vi "量测站CT内容.vi"() -> (0 "tablename":string, 3 "data":string[](array[string]))   [LabVIEW 2017]
uses:
  Sqlite/CBB/ReadAllData.vi
  Sqlite/SQLite.lvlib
panel:
  out "大小 2":i32
  out "大小":i32
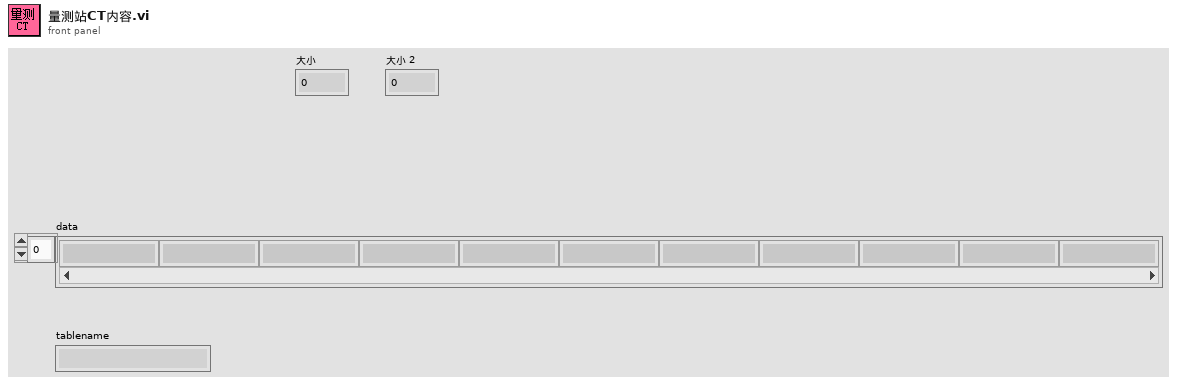
[diagram p1: front panel]
types:
  T1 = typedef "动子1&2CT操作选项.ctl" = enum16{"初始化", "出料轴接料", "投掷出料区", "获取寄存器", "更新等待CT"}
  T2 = typedef "动子3&4CT操作选项.ctl" = enum16{"初始化", "扫码+CheckRoute", "BK拍照", "BT+对位", "RT贴合", "Servo压合", "p400复检", "获取寄存器", "更新等待时间"}
  T3 = typedef "data格式选项.ctl" = enum16{"生成格式", "加载格式"}
  T4 = typedef "pathcheck选项.ctl" = enum16{"ProductData", "CTData", "ERData", "IOTDATA"}
  T5 = typedef "IOT time.ctl" = cluster{"Work":string, "Inflow":string, "Outflow":string, "Wait":string}
  T6 = typedef "上一次缓存.ctl" = cluster{"CT集合":string[], "in /out time":T7, "SN缓存":string}
  T7 = typedef "in_out time.ctl" = cluster{"input-time":string, "output-time":string, "wait-starttime":dbl, "wait-time":string}
  T8 = typedef "表头集合.ctl" = cluster{"product信息":T9, "CT信息":T10, "ER信息":T11, "IOT信息":T12}
  T9 = typedef "product信息.ctl" = cluster{"product表头整合":string[], "量测部分表头":string[], "前侧贴合表头":string[], "后侧贴合表头":string[]}
  T10 = typedef "CT信息.ctl" = cluster{"CT表头整合":string[], "量测CT":string[], "动子1_2CT":string[], "动子3_4CT":string[]}
  T11 = typedef "ER信息.ctl" = cluster{"ER表头整合":string[]}
  T12 = typedef "IOT信息.ctl" = cluster{"IOT表头整合":string[]}
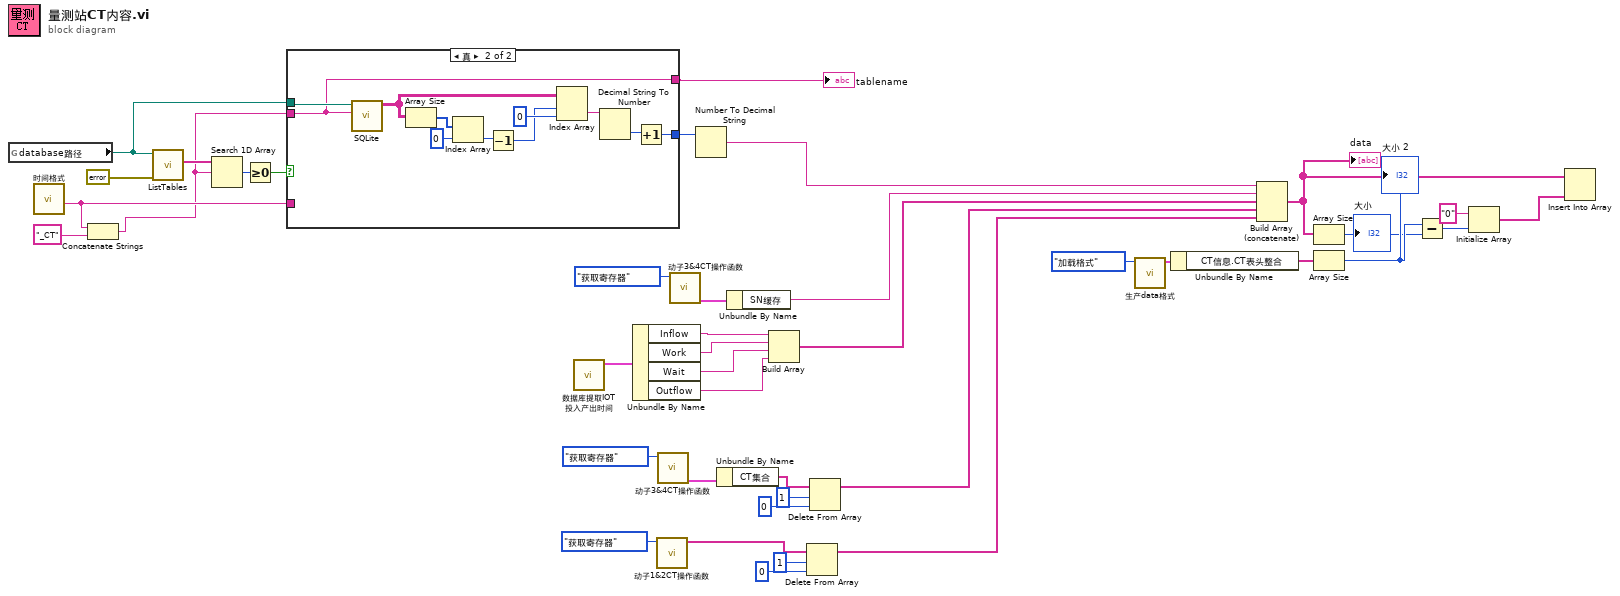
[diagram p0: block diagram]
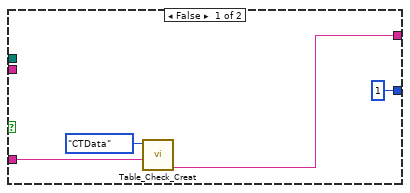
[diagram p2: hidden frame]
diagram:
  n1 = global read "数据库全局.vi" "database路径"() -> (w27:path)
  n2 = call "时间格式.vi"() -> ("_Date"=w25:string)  [unwired: 7 in, 4 out]
  n3 = Concatenate Strings(w25, "_CT" ("字符串")) -> (w24:string)
  n4 = call "ListTables.vi"("error in (no error)"=errorcluster {"status"=FALSE, "code"=0, "source"=""}, "DbPath"=w27) -> ("Tables"=w30:string[])  [unwired: 6 in, 3 out]
  n5 = Search 1D Array(1D array=w30, element=w24) -> (index of element=w31:i32)  [unwired: 1 in]
  n6 = Greater Or Equal To 0?(x=w31) -> (x >= 0?=w28:bool)
  n7 = case shown="真" w28 {
    tunnel: w27 -> [_ w55]
    tunnel: w24 -> [_ w45]
    tunnel: [1 w46] -> w26
    tunnel: w25 -> [w42 _]
    tunnel: [w41 w45] -> w23
    frame False {
      n8 = call "Table_Check_Creat.vi"("_datetime"=w42, "pathcheck选项"=pathcheck选项."CTData") -> ("tablename"=w41:string)  [unwired: 7 in, 2 out]
    }
    frame True {
      n9 = call-poly "SQLite.vi"("Table Name"=w45, "DbPath"=w55) -> ("Results"=w53:string[][])  [unwired: 4 in, 5 out]
      n10 = Array Size(array=w53) -> (size(s)=w52:i32[])
      n11 = Index Array(array=w52, index=0 ("索引")) -> (element=w50:i32)
      n12 = Decrement(x=w50) -> (x-1=w49:i32)
      n13 = Index Array(array=w53, index (row)=w49, index (col)=0 ("禁用的索引 (列)")) -> (element=w48:string)
      n14 = Decimal String To Number(string=w48) -> (number=w47:i32)  [unwired: 2 in, 1 out]
      n15 = Increment(x=w47) -> (x+1=w46:i32)
    }
  }
  "tablename" <- w23
  n16 = call "数据库提取IOT 投入产出时间.vi"() -> ("IOT time"=w18:T5)  [unwired: 11 in]
  n17 = Unbundle By Name(w18) -> ("Inflow"=w17:string, "Work"=w16:string, "Wait"=w15:string, "Outflow"=w14:string)
  n18 = call "动子1&2CT操作函数.vi"("CT操作选项"=动子1&2CT操作选项."获取寄存器") -> ("CT集合"=w3:string[])  [unwired: 9 in, 1 out]
  n19 = call "动子3&4CT操作函数.vi"("CT操作选项"=动子3&4CT操作选项."获取寄存器") -> ("上一次缓存"=w10:T6)  [unwired: 8 in, 2 out]
  n20 = call "动子3&4CT操作函数.vi"("CT操作选项"=动子3&4CT操作选项."获取寄存器") -> ("上一次缓存"=w20:T6)  [unwired: 8 in, 2 out]
  n21 = Number To Decimal String(number=w26) -> (decimal integer string=w22:string)  [unwired: 1 in]
  n22 = Unbundle By Name(w10) -> ("CT集合"=w9:string[])
  n23 = Unbundle By Name(w20) -> ("SN缓存"=w19:string)
  n24 = Build Array(w17, w16, w15, w14) -> (w13:string[])
  n25 = Delete From Array(array=w3, length=1 ("长度"), index=0 ("长度")) -> (array with subset deleted=w2:string[])  [unwired: 1 out]
  n26 = Delete From Array(array=w9, length=1 ("长度"), index=0 ("长度")) -> (array with subset deleted=w6:string[])  [unwired: 1 out]
  n27 = call "生产data格式.vi"("data格式选项"=data格式选项."加载格式") -> ("表头格式"=w39:T8)  [unwired: 10 in]
  n28 = Unbundle By Name(w39) -> ("CT信息.CT表头整合"=w38:string[])
  n29 = Build Array (concatenate)(w22, w19, w13, w6, w2) -> (w1:string[])
  "data" <- w1
  n30 = Array Size(array=w1) -> (size(s)=w36:i32)
  "大小" <- w36
  n31 = Array Size(array=w38) -> (size(s)=w37:i32)
  "大小 2" <- w37
  n32 = Subtract(x=w37, y=w36) -> (x-y=w35:i32)
  n33 = Initialize Array("0", w35) -> (w33:string[])
  n34 = Insert Into Array(array=w1, new element=w33) -> ()  [unwired: 1 in, 1 out]
